vi "Webcam grab example 2.vi"() -> ()   [LabVIEW 2013]
doc: "The Low-Level Grab Raw Data VI acquires images continuously using low-level acquisition VIs. This VI demonstrates how to acquire raw data from the camera. A grab is appropriate for high-speed applications in which you need to process only one image at a time."
panel:
  out "Tube":i16[][](graph)
  out "Bird":i16[][](graph)
  out "Green":i16[][](graph)
  out "Blue":i16[][](graph)
  out "Red":i16[][](graph)
  out "Image Pixels (U32)":u32[][](graph)
  in  "Camera Name":refnum<k21> caption="IMAQdx Session"
  in  "Stop":bool
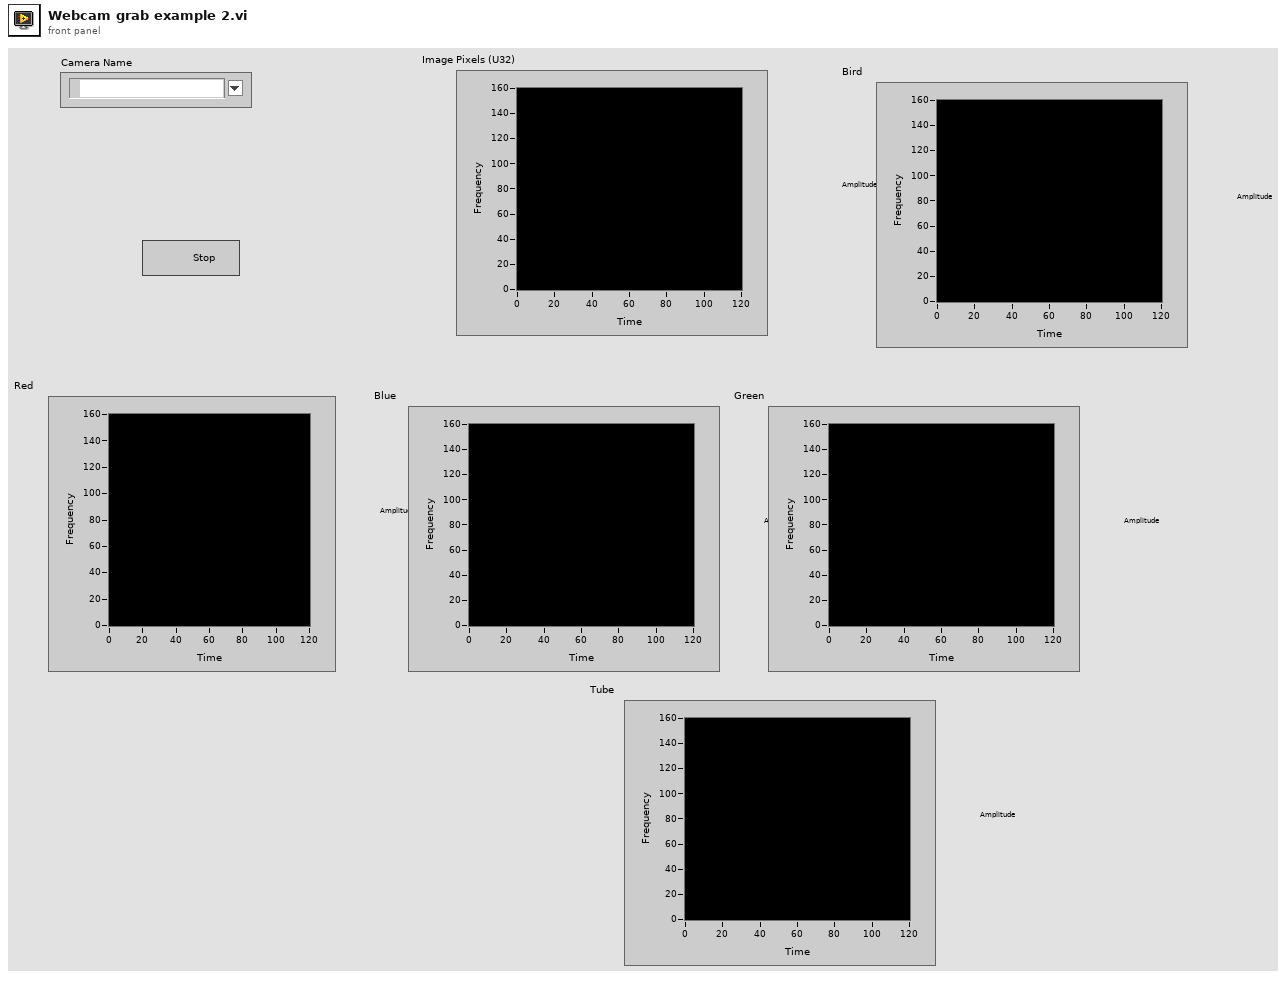
[diagram p1: front panel]
types:
  T1 = typedef "IMAQ Image.ctl" = refnum<image>
  T2 = typedef "IMAQdx.ctl" = refnum<k21>
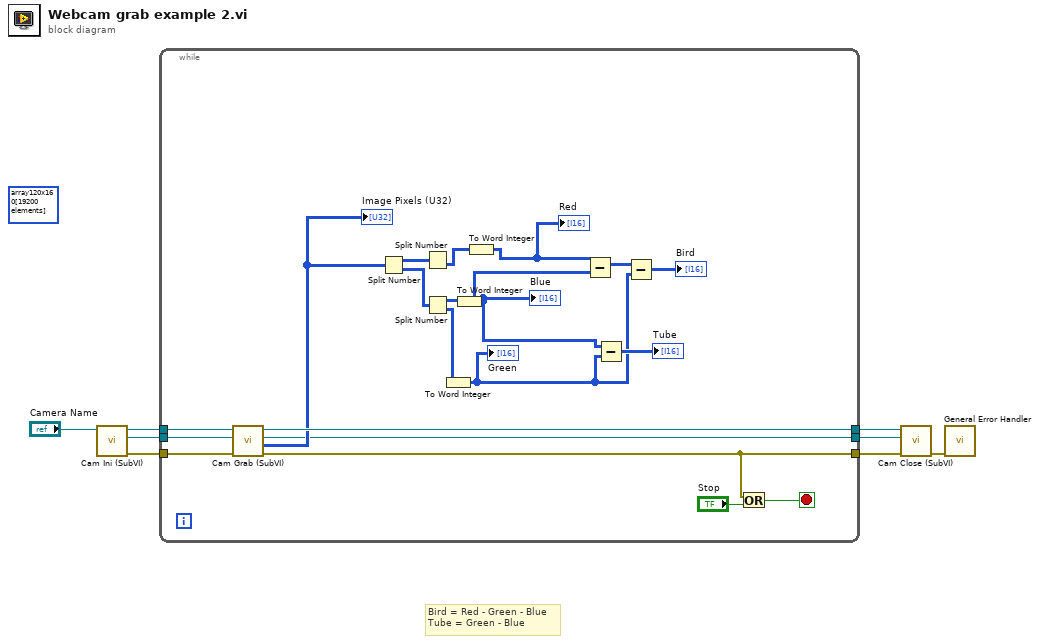
[diagram p0: block diagram]
diagram:
  (unwired) u32[][] array120x160[19200 elements] ("Image Pixels (U32)")
  # "Bird = Red - Green - Blue\nTube = Green - Blue"
  n1 = call "Cam Ini (SubVI).vi"("Camera"="Camera Name") -> ("error out"=w7:errorcluster, "Image Ref"=w3:T1, "Cam Ref"=w6:T2)  [unwired: 8 in]
  n2 = while {
    tunnel: [w25] -> w2
    tunnel: w7 -> [w26]
    tunnel: w6 -> [w12]
    tunnel: [w24] -> w5
    tunnel: w3 -> [w11]
    tunnel: [w9] -> w1
    stop <- w28 stop-if-true
    n3 = call "Cam Grab (SubVI).vi"("error in (no error)"=w26, "Refnum in"=w11, "Cam Ref"=w12) -> ("error out"=w24:errorcluster, "Image Pixels (U32)"=w10:u32[][], "Refnum dup"=w9:T1, "Refnum out"=w25:T2)  [unwired: 5 in]
    "Image Pixels (U32)" <- w10
    n4 = Split Number(x=w10) -> (hi(x)=w23:u16[][], lo(x)=w22:u16[][])
    n5 = Split Number(x=w23) -> (lo(x)=w18:u8[][])  [unwired: 1 out]
    n6 = Split Number(x=w22) -> (hi(x)=w16:u8[][], lo(x)=w14:u8[][])
    n7 = To Word Integer(number=w14) -> (16bit integer=w13:i16[][])
    "Green" <- w13
    n8 = To Word Integer(number=w16) -> (16bit integer=w15:i16[][])
    "Blue" <- w15
    n9 = To Word Integer(number=w18) -> (16bit integer=w17:i16[][])
    "Red" <- w17
    n10 = Subtract(x=w17, y=w15) -> (x-y=w21:i16[][])
    n11 = Subtract(x=w15, y=w13) -> (x-y=→"Tube":i16[][])
    n12 = Subtract(x=w21, y=w13) -> (x-y=→"Bird":i16[][])
    n13 = Or(x=w24, y="Stop") -> (x .or. y?=w28:bool)
  }
  n14 = call "Cam Close (SubVI).vi"("error in (no error)"=w5, 10:"Refnum in"=w1, 11:"Refnum in"=w2) -> ("error out"=w8:errorcluster)  [unwired: 8 in]
  n15 = call <vilib>:"General Error Handler.vi"("error in (no error)"=w8) -> ()  [unwired: 1 in, 14 out]
